vi "Check Vacuum Level.vi"(7 "Vacuum Specs":T1, 8 "error in (no error)":errorcluster) -> (0 "error out":errorcluster, 3 "Array":T2[](array[typedef]))   [LabVIEW 2018]
uses:
  Vacuum Test.ctl
  Vacuum Specs.ctl
  Hardware/DAQ Mngr.ctl
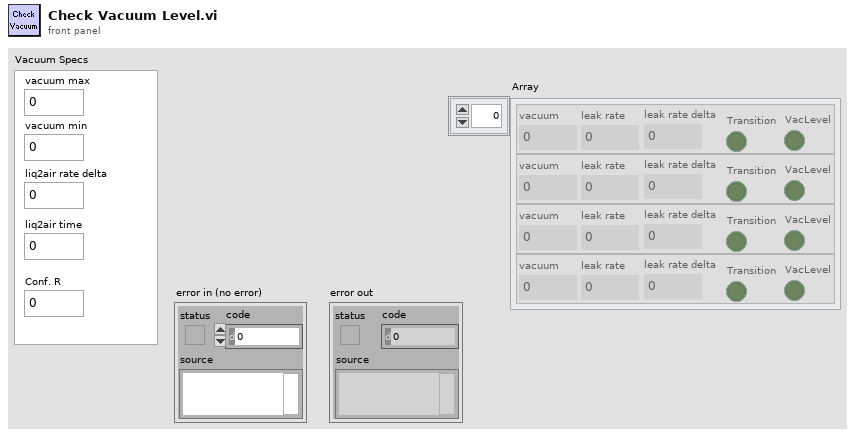
[diagram p1: front panel]
types:
  T1 = typedef "Vacuum Specs.ctl" = cluster{"vacuum max":dbl, "vacuum min":dbl, "liq2air rate delta":dbl, "liq2air time":dbl, "Conf. R":dbl}
  T2 = typedef "Vacuum Test.ctl" = cluster{"Transition":bool, "VacLevel":bool, "leak rate":dbl, "vacuum":dbl, "leak rate delta":dbl}
  T3 = typedef "DAQ Mngr.ctl" = enum16{"Init", "Read Vacuum", "Analyze Vacuum", "Read Cartridges", "Lock Cartridge", "Unlock Cartridge", "Read PS", "Close"}
  T4 = typedef "Vacuum Output.ctl" = cluster{"Vacuum":dbl, "Rate":dbl, "R":dbl}
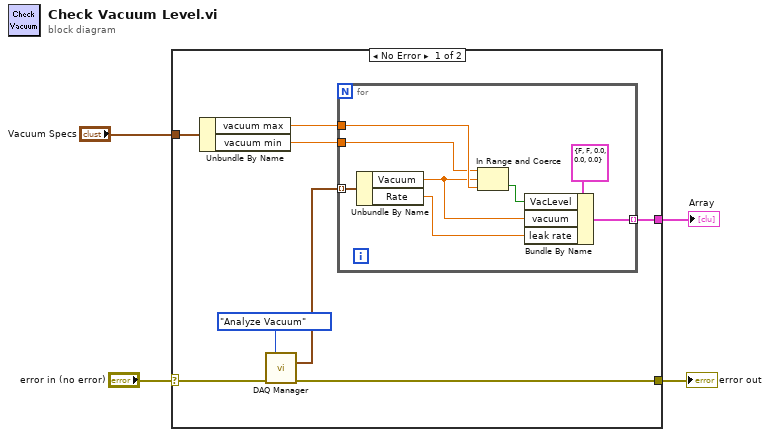
[diagram p0: block diagram]
diagram:
  n1 = case shown="No Error" "error in (no error)" {
    selector: "error in (no error)" -> [w11 w21]
    tunnel: [w8 w21] -> w3
    tunnel: "Vacuum Specs" -> [w6 _]
    tunnel: [w5 _] -> w1
    frame No Error {
      n2 = Unbundle By Name(w6) -> ("vacuum max"=w9:dbl, "vacuum min"=w10:dbl)
      n3 = call "DAQ Manager.vi"("DAQ Mngr Action"=DAQ_Mngr."Analyze Vacuum", "error in (no error)"=w11) -> ("Data Array"=w7:T4[], "error out"=w8:errorcluster)  [unwired: 8 in, 4 out]
      n4 = for {
        tunnel: w9 -> [w20]
        tunnel: w10 -> [w19]
        tunnel: [w16] -> w5 mode=indexing
        tunnel: w7 -> [w13] mode=indexing
        n5 = Unbundle By Name(w13) -> ("Vacuum"=w14:dbl, "Rate"=w15:dbl)
        n6 = In Range and Coerce(upper limit=w19, x=w14, lower limit=w20) -> (In Range?=w17:bool)  [unwired: 1 out]
        n7 = Bundle By Name(cluster=T2 {"Transition"=FALSE, "VacLevel"=FALSE, "leak rate"=0.0, "vacuum"=0.0, "leak rate delta"=0.0} ("Result"), "VacLevel"=w17, "vacuum"=w14, "leak rate"=w15) -> (w16:T2)
      }
    }
    frame Error {
    }
  }
  "error out" <- w3
  "Array" <- w1
